vi "formatAmountToCellInterface.vi"(8 "error in (no error)":errorcluster, 11 "UserEditableAmount in":refnum<class "UserEditableAmount.lvclass">) -> (0 "error out":errorcluster, 2 "Cell Interface":string, 3 "UserEditableAmount out":refnum<class "UserEditableAmount.lvclass">)   [LabVIEW 2018, in "UserEditableAmount.lvclass"]
uses:
  UserEditableAmount.lvclass
  UserEditableAmount.lvclass/UserEditableAmount.ctl
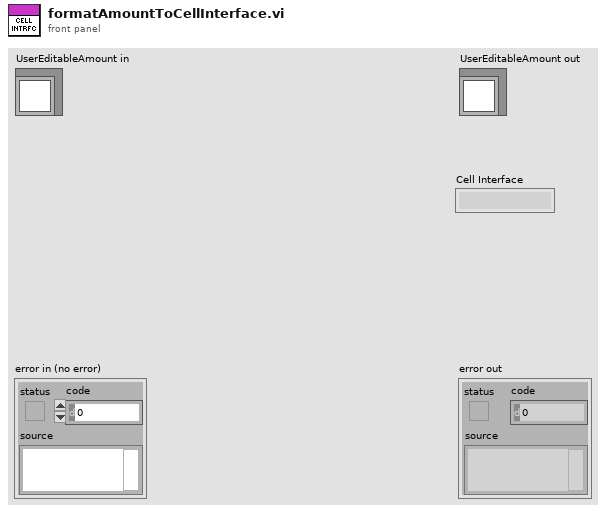
[diagram p1: front panel]
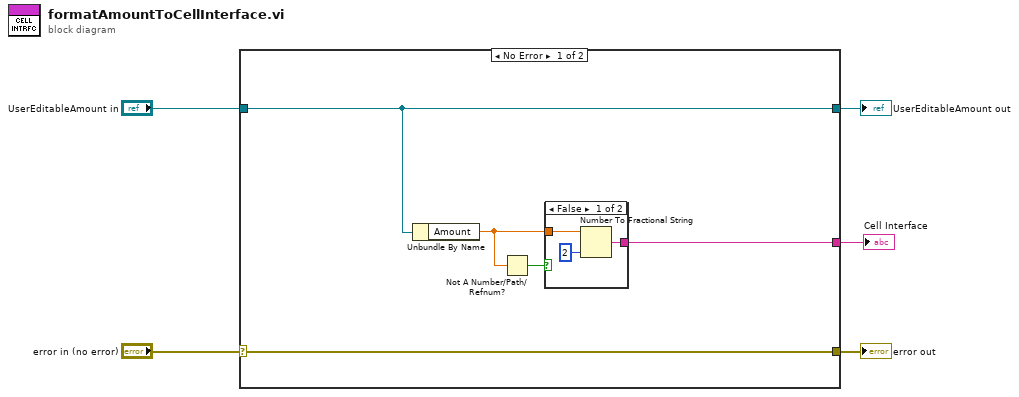
[diagram p0: block diagram]
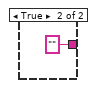
[diagram p2: hidden frame]
diagram:
  n1 = case shown="No Error" "error in (no error)" {
    selector: "error in (no error)" -> [w10 w16]
    tunnel: [w10 w16] -> w4
    tunnel: [w8 w15] -> w2
    tunnel: "UserEditableAmount in" -> [w8 w15]
    tunnel: [w6 _] -> w1
    frame No Error {
      n2 = Unbundle By Name(w8) -> ("Amount"=w7:dbl)
      n3 = Not A Number/Path/Refnum?(number/path/refnum=w7) -> (NaN/Path/Refnum?=w9:bool)
      n4 = case shown="False" w9 {
        tunnel: [w12 ""] -> w6
        tunnel: w7 -> [w11 _]
        frame False {
          n5 = Number To Fractional String(number=w11, precision (6)=i16 2) -> (F-format string=w12:string)  [unwired: 2 in]
        }
        frame True {
        }
      }
    }
    frame Error {
    }
  }
  "error out" <- w4
  "UserEditableAmount out" <- w2
  "Cell Interface" <- w1
